vi "shuffle.vi"(1 "Array IN":variant[][](array[variant])) -> (0 "Array OUT":variant[][](array[variant]))   [LabVIEW 2015, in "oskar_tools.lvlib"]
uses:
  oskar_tools.lvlib
panel:
  out "size(s)":i32[](array[numeric])
  out "element":i32
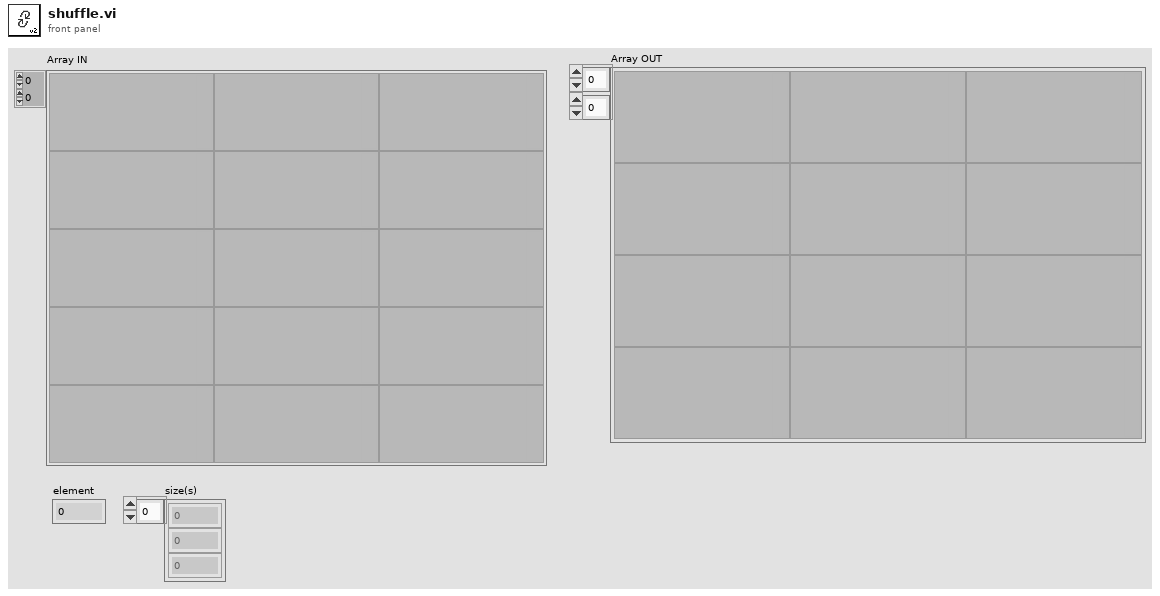
[diagram p1: front panel]
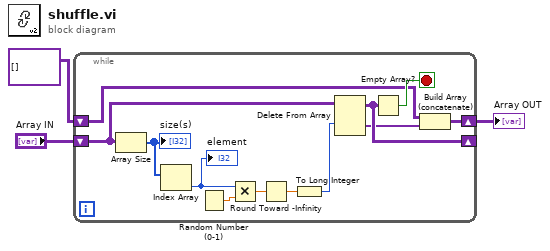
[diagram p0: block diagram]
diagram:
  n1 = while {
    shift-right: [w15] -> _
    shift-left: "Array IN" -> [w13]
    shift-right: [w9] -> w2
    shift-left: variant[][] [] -> [w11]
    stop <- w14 stop-if-true
    n2 = Array Size(array=w13) -> (size(s)=w4:i32[])
    "size(s)" <- w4
    n3 = Index Array(array=w4) -> (element=w5:i32)  [unwired: 1 in]
    "element" <- w5
    n4 = Random Number (0-1)() -> (number: 0 to 1=w12:dbl)
    n5 = Multiply(x=w5, y=w12) -> (x*y=w8:dbl)
    n6 = Round Toward -Infinity(1:w8) -> (0:w7:dbl)
    n7 = To Long Integer(number=w7) -> (32bit integer=w6:i32)
    n8 = Delete From Array(array=w13, index (row)=w6) -> (deleted portion=w10:variant[], array with subset deleted=w15:variant[][])  [unwired: 2 in]
    n9 = Empty Array?(array=w15) -> (empty?=w14:bool)
    n10 = Build Array (concatenate)(w11, w10) -> (w9:variant[][])
  }
  "Array OUT" <- w2
